vi "DDS_serialProgrammer.vi"(0 "Device In":T2={"Device Description"="", "Handle"=-1}, 1 "Reinitialize DDS":bool, 5 "Characters to FPGA":string="L;004\r\nL102200242\r\nL2000034\r\nL01\r\nL411<71<720::::::;0::::::;071<71<7\r\nL615555555155555550>38>38>0>38>38>\r\nL31000100010001000\r\nL50000000000000000\r\nL70200000001010000000102000000010200000001\r\nL80200000001010000000102000000010200000001\r\nL:0;>;<2000;>;<2000;>;<2000;>;<200\r\nL91010\r\n", 11 "error in":errorcluster) -> (4 "Device Out":T1={"Device Description"="Ultracool FPGA 03", "Handle In"=-1}, 6 "Bytes Written":u32=278, 8 "FT_Status":u32(ring) items=["FT_OK", "FT_INVALID_HANDLE", "FT_DEVICE_NOT_FOUND", "FT_DEVICE_NOT_OPENED", "FT_IO_ERROR", "FT_INSUFFICIENT_RESOURCES", "FT_INVALID_PARAMETER", "FT_INVALID_BAUD_RATE", "FT_DEVICE_NOT_OPENED_FOR_ERASE", "FT_DEVICE_NOT_OPENED_FOR_WRITE", "FT_FAILED_TO_WRITE_DEVICE", "FT_EEPROM_READ_FAILED", "FT_EEPROM_WRITE_FAILED", "FT_EEPROM_ERASE_FAILED", "FT_EEPROM_NOT_PRESENT", "FT_EEPROM_NOT_PROGRAMMED", "FT_INVALID_ARGS", "FT_NOT_SUPPORTED", "FT_OTHER_ERROR"], 10 "Characters written to FPGA":string, 15 "error out":errorcluster)   [LabVIEW 2013, in "DDS9954_v2013.lvlib"]
uses:
  DDS9954_v2013.lvlib
panel:
  out "Handle Out":i64
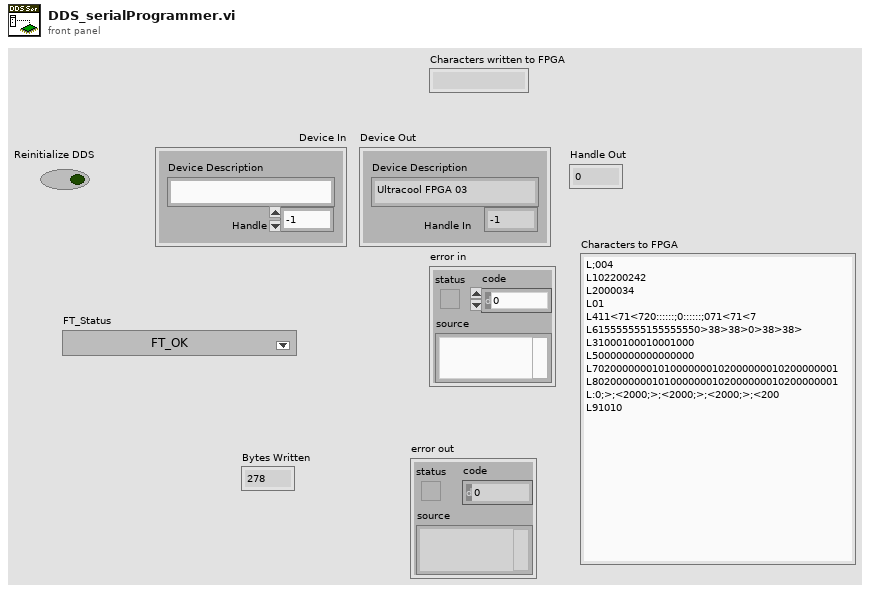
[diagram p1: front panel]
types:
  T1 = cluster{"Device Description":string, "Handle In":i64}
  T2 = cluster{"Device Description":string, "Handle":i64}
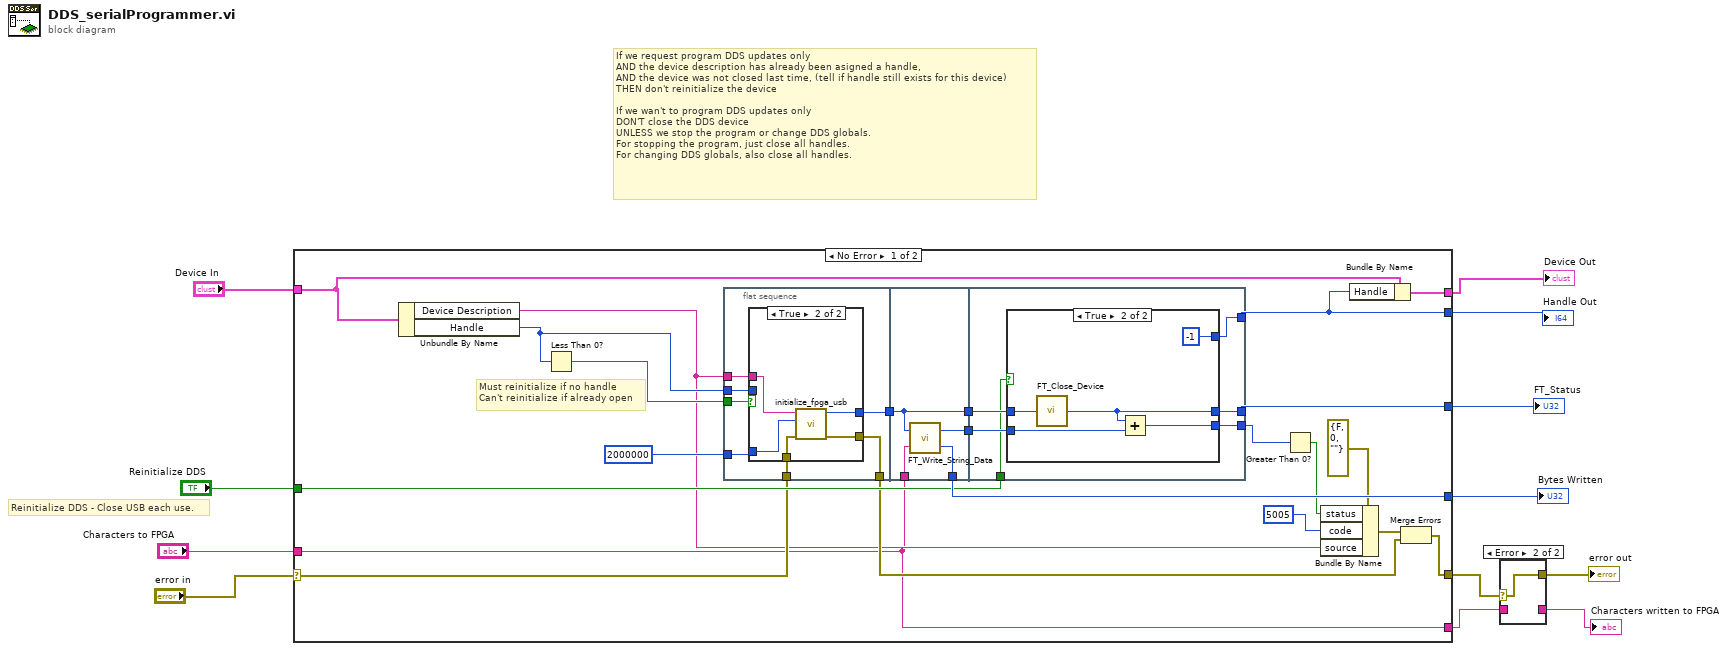
[diagram p0: block diagram]
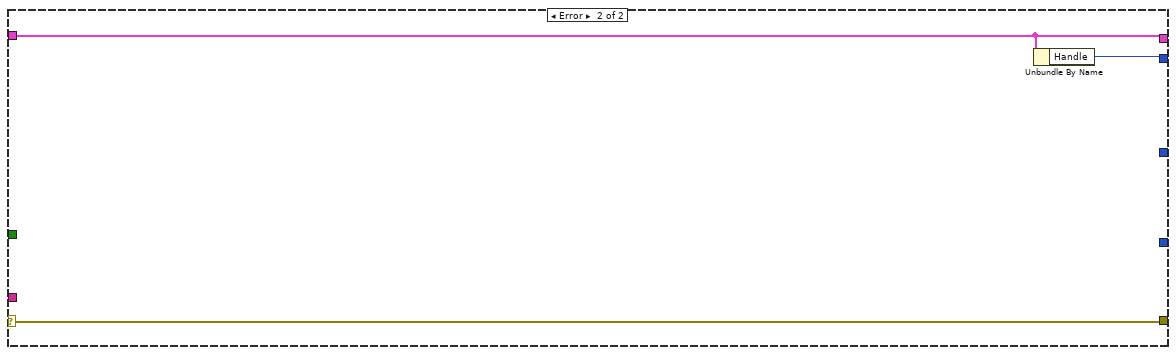
[diagram p5: hidden frame]
diagram:
  # "Reinitialize DDS - Close USB each use."
  # "If we request program DDS updates only\nAND the device description has already been asigned a handle,\nAND the device was not closed last time, (tell if handle still exists for this device)\nTHEN don't reinitialize the device\n\nIf we wan't to program DDS updates only\nDON'T close the DDS device\nUNLESS we stop the program or change DDS globals.\nFor stopping the program, just close all handles.\nFor changing DDS globals, also close all handles."
  n1 = case shown="No Error" "error in" {
    selector: "error in" -> [w25 w66]
    tunnel: "Characters to FPGA" -> [w13 _]
    tunnel: [w31 _] -> w11
    tunnel: [w30 _] -> w10
    tunnel: [w19 w66] -> w4
    tunnel: "Device In" -> [w14 w68]
    tunnel: [w16 w67] -> w8
    tunnel: "Reinitialize DDS" -> [w26 _]
    tunnel: [w15 w68] -> w5
    tunnel: [w13 _] -> w3
    frame No Error {
      # "Must reinitialize if no handle\nCan't reinitialize if already open"
      n2 = Unbundle By Name(w14) -> ("Device Description"=w18:string, "Handle"=w28:i64)
      n3 = Less Than 0?(x=w28) -> (x < 0?=w27:bool)
      n4 = flat-sequence {
        tunnel: [w41] -> w34
        tunnel: w18 -> [w40]
        tunnel: u32 2000000 ("Baud Rate") -> [w39]
        tunnel: [w38] -> w20
        tunnel: w27 -> [w37]
        tunnel: w28 -> [w36]
        tunnel: w25 -> [w35]
        tunnel: w34 -> [w49]
        tunnel: [w52] -> w31
        tunnel: w13 -> [w51]
        tunnel: [w49] -> w33
        tunnel: [w50] -> w32
        tunnel: w33 -> [w58]
        tunnel: [w57] -> w30
        tunnel: w32 -> [w56]
        tunnel: [w55] -> w24
        tunnel: [w54] -> w16
        tunnel: w26 -> [w53]
        frame #0 {
          n5 = case shown="True" w37 {
            tunnel: [w43 w48] -> w41
            tunnel: w40 -> [_ w47]
            tunnel: w39 -> [_ w46]
            tunnel: [w42 w45] -> w38
            tunnel: w36 -> [w43 _]
            tunnel: w35 -> [w42 w44]
            frame False {
            }
            frame True {
              n6 = call "initialize_fpga_usb.vi"("error in"=w44, "Baud Rate"=w46, "Device Description"=w47) -> ("error out"=w45:errorcluster, "Handle"=w48:u32)  [unwired: 3 in]
            }
          }
        }
        frame #1 {
          n7 = call "FT_Write_String_Data.vi"("Buffer"=w51, "Handle"=w49) -> ("Bytes Written"=w52:u32, "FT_Status"=w50:u32)
        }
        frame #2 {
          n8 = case shown="True" w53 {
            tunnel: w58 -> [w60 w65]
            tunnel: [w59 w64] -> w57
            tunnel: w56 -> [w59 w63]
            tunnel: [w59 w62] -> w55
            tunnel: [w60 i64 -1 ("Handle In")] -> w54
            frame False {
            }
            frame True {
              n9 = call "FT_Close_Device.vi"("Handle"=w65) -> ("FT_Status"=w64:u32)
              n10 = Add(x=w64, y=w63) -> (x+y=w62:u32)
            }
          }
        }
      }
      n11 = Greater Than 0?(x=w24) -> (x > 0?=w17:bool)
      n12 = Bundle By Name(cluster=errorcluster {"status"=FALSE, "code"=0, "source"=""} ("error constant"), "status"=w17, "code"=5005, "source"=w18) -> (w23:errorcluster)
      n13 = Bundle By Name(cluster=w14, "Handle"=w16) -> (w15:T2)
      n14 = Merge Errors(w23, w20) -> (w19:errorcluster)
    }
    frame Error {
      n15 = Unbundle By Name(w68) -> ("Handle"=w67:i64)
    }
  }
  "Bytes Written" <- w11
  "FT_Status" <- w10
  "Handle Out" <- w8
  "Device Out" <- w5
  n16 = case shown="Error" w4 {
    selector: w4 -> [w69 w71]
    tunnel: w3 -> [w70 _]
    tunnel: [w70 _] -> w2
    tunnel: [w69 w71] -> w1
    frame No Error {
    }
    frame Error {
    }
  }
  "error out" <- w1
  "Characters written to FPGA" <- w2
